vi "UDP_SendReceive_LV.vi"() -> ()   [LabVIEW 2020]
uses:
  LV2Py.ctl
  Py2LV.ctl
panel:
  out "Py2LV":T1
  in  "LV2Py":T2
  in  "Stop":bool
  # "This boolean will stop python console and exit out the console."
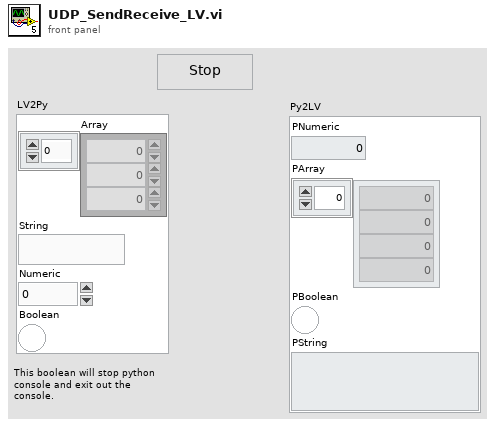
[diagram p1: front panel]
types:
  T1 = typedef "Py2LV.ctl" = cluster{"PNumeric":dbl, "PArray":dbl[], "PBoolean":bool, "PString":string}
  T2 = typedef "LV2Py.ctl" = cluster{"Array":dbl[], "String":string, "Numeric":i32, "Boolean":bool}
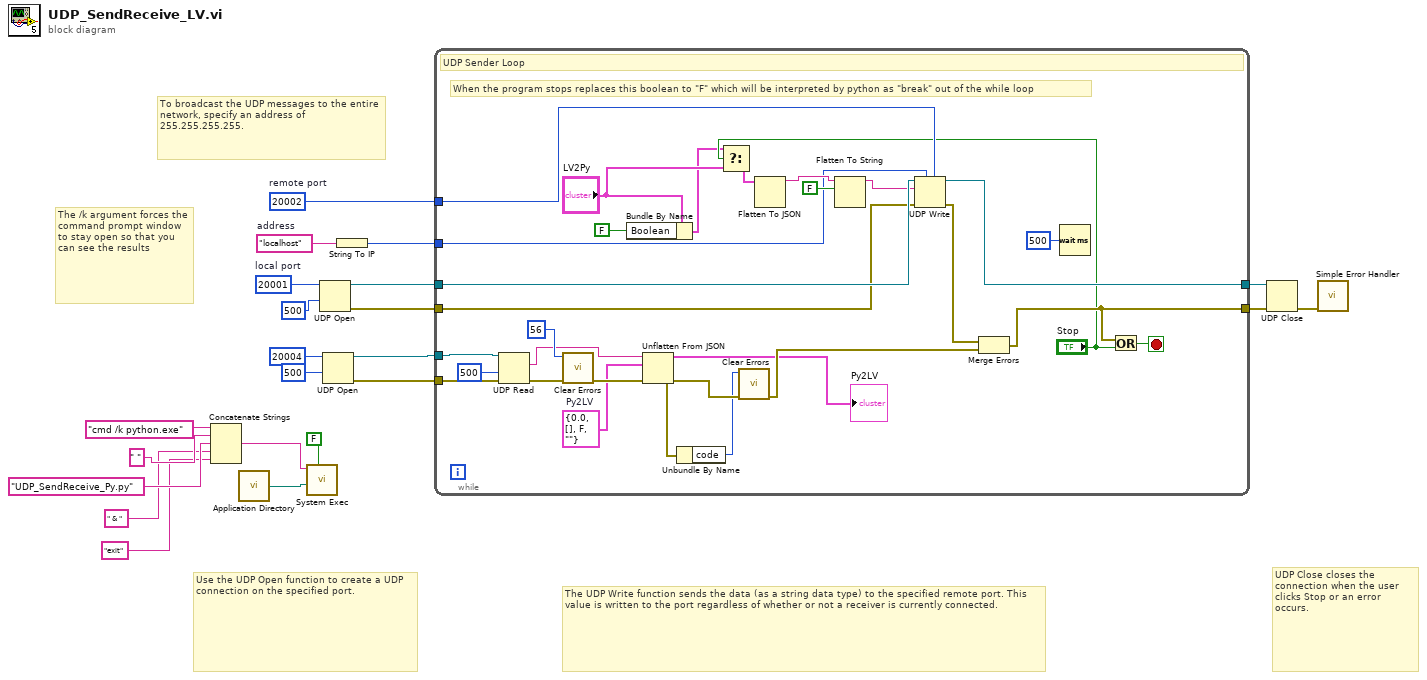
[diagram p0: block diagram]
diagram:
  w14 = u16 20002  # remote port
  w15 = u16 20001  # local port
  w20 = "localhost"  # address
  # "The /k argument forces the command prompt window to stay open so that you can see the results"
  # "To broadcast the UDP messages to the entire network, specify an address of 255.255.255.255."
  # "UDP Close closes the connection when the user clicks Stop or an error occurs."
  # "The UDP Write function sends the data (as a string data type) to the specified remote port. This value is written to the port regardless of whether or not a receiver is currently connected."
  # "Use the UDP Open function to create a UDP connection on the specified port."
  n1 = Concatenate Strings("cmd /k python.exe" ("string"), " " ("string"), "UDP_SendReceive_Py.py" ("string"), " & " ("string"), "exit" ("string")) -> (w9:string)
  n2 = call <vilib>:"Application Directory.vi"() -> ("Application Directory"=w5:path)
  n3 = call <vilib>:"System Exec.vi"("wait until completion? (T)"=FALSE, "working directory"=w5, "command line"=w9) -> ()  [unwired: 5 in, 4 out]
  n4 = UDP Open(9:500 ("timeout ms (25000)"), 11:w15) -> (port=w17:refnum<k16>, 0:w16:errorcluster)  [unwired: 3 in, 1 out]
  n5 = UDP Open(9:500 ("timeout ms (25000)"), 11:u16 20004 ("port")) -> (port=w13:refnum<k16>, 0:w12:errorcluster)  [unwired: 3 in, 1 out]
  n6 = String To IP(1:w20) -> (0:w18:u32)
  n7 = while {
    tunnel: [w36] -> w21
    tunnel: w17 -> [w51]
    tunnel: w16 -> [w50]
    tunnel: [w48] -> w22
    tunnel: w18 -> [w23]
    tunnel: w14 -> [w46]
    tunnel: w13 -> [w42]
    tunnel: w12 -> [w41]
    stop <- w49 stop-if-true
    w24 = T1 {"PNumeric"=0.0, "PArray"=[], "PBoolean"=FALSE, "PString"=""}  # Py2LV
    # "When the program stops replaces this boolean to \"F\" which will be interpreted by python as \"break\" out of the while loop"
    # "UDP Sender Loop"
    n8 = UDP Read(connection ID=w42, timeout ms (25000)=500, 8:w41) -> (data out=w37:string, error out=w40:errorcluster)  [unwired: 4 out]
    n9 = call <vilib>:"Clear Errors.vi"("error in (no error)"=w40, "specific error code to clear (0: all)"=56) -> ("error out"=w28:errorcluster)  [unwired: 4 in, 1 out]
    n10 = Bundle By Name(cluster="LV2Py", "Boolean"=FALSE) -> (w33:T2)
    n11 = Unflatten From JSON(JSON string=w37, type and defaults=w24, error in (no error)=w28) -> (value=→"Py2LV":T1, error out=w27:errorcluster)  [unwired: 4 in]
    n12 = Unbundle By Name(w27) -> ("code"=w26:i32)
    n13 = Select(t=w33, s="Stop", f="LV2Py") -> (s? t:f=w32:T2)
    n14 = call <vilib>:"Clear Errors.vi"("error in (no error)"=w27, "specific error code to clear (0: all)"=w26) -> ("error out"=w29:errorcluster)  [unwired: 4 in, 1 out]
    n15 = Flatten To JSON(anything=w32) -> (JSON string=w45:string)  [unwired: 2 in, 1 out]
    n16 = Flatten To String(anything=w45, prepend array or string size? (T)=FALSE) -> (data string=w44:string)  [unwired: 2 in, 2 out]
    n17 = UDP Write(address=w23, port or service name=w46, connection ID=w51, data in=w44, 8:w50) -> (error out=w38:errorcluster, 3:w48:refnum<k16>)  [unwired: 1 in]
    n18 = Merge Errors(w38, w29) -> (w36:errorcluster)
    n19 = Wait (ms)(milliseconds to wait=u32 500) -> ()  [unwired: 1 out]
    n20 = Or(x=w36, y="Stop") -> (x .or. y?=w49:bool)
  }
  n21 = UDP Close(connection ID=w22, 8:w21) -> (error out=w19:errorcluster)  [unwired: 1 out]
  n22 = call <vilib>:"Simple Error Handler.vi"("error in (no error)"=w19) -> ()  [unwired: 4 in, 5 out]
